vi "CRYReport Pic LIB.vi"(6 "sOption":string, 7 "sAction":string, 8 "nData":i32, 9 "sData":string, 10 "cView":T2, 11 "cFrame":T1) -> (0 "nData_Out":i32, 1 "sData_Out":string, 2 "cView_Out":T2, 3 "cFrame_Out":T1)   [LabVIEW 2013]
uses:
  CRYReport Global.vi
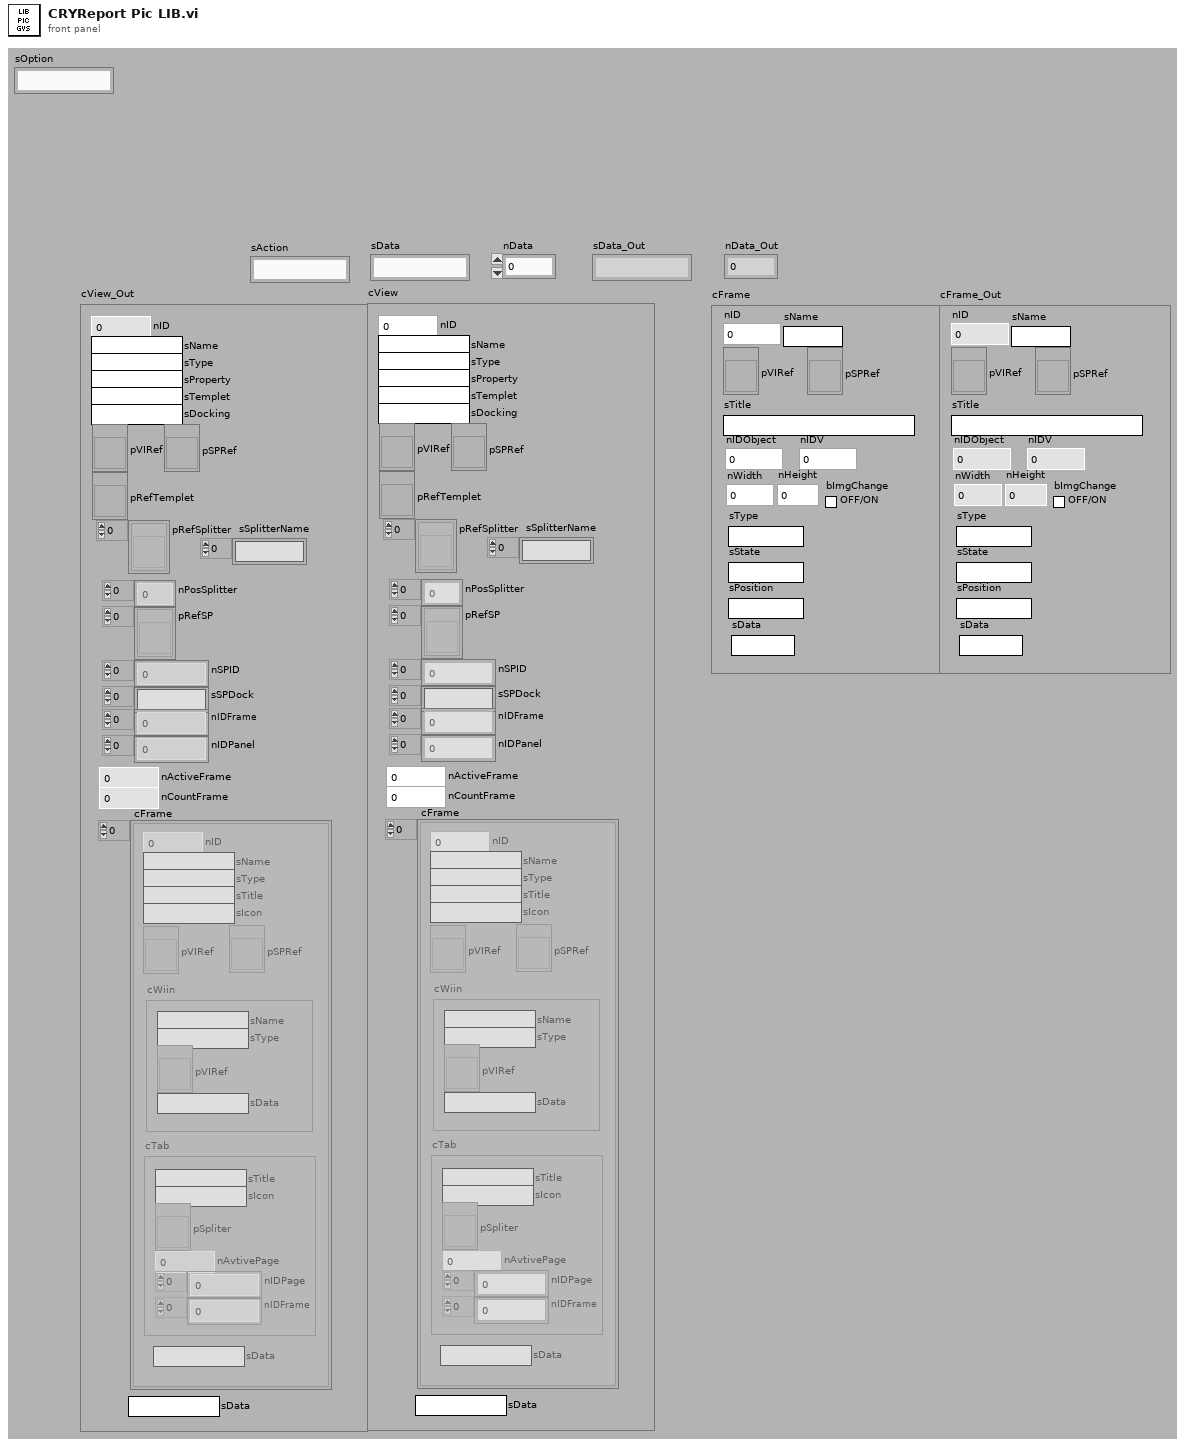
[diagram p1: front panel]
types:
  T1 = cluster{"nID":i16, "sName":string, "pVIRef":refnum<vi>, "pSPRef":refnum<vi>, "sTitle":string, "nIDObject":i16, "nIDV":i16, "nWidth":i16, "nHeight":i16, "bImgChange":bool, "sType":string, "sState":string, "sPosition":string, "sData":string}
  T2 = cluster{"nID":i32, "sName":string, "sType":string, "sProperty":string, "sTemplet":string, "sDocking":string, "pVIRef":refnum<vi>, "pSPRef":refnum<vi>, "pRefTemplet":refnum<vi>, "pRefSplitter":refnum<vi>[], "nPosSplitter":i32[], "pRefSP":refnum<vi>[], "nSPID":i32[], "sSPDock":string[], "nIDFrame":i32[], "nIDPanel":i32[], "nActiveFrame":i32, "nCountFrame":i32, "cFrame":cluster{"nID":i32, "sName":string, "sType":string, "sTitle":string, "sIcon":string, "pVIRef":refnum<vi>, "pSPRef":refnum<vi>, "cWiin":cluster{"sName":string, "sType":string, "pVIRef":refnum<vi>, "sData":string}, "cTab":cluster{"sTitle":string, "sIcon":string, "pSpliter":refnum<vi>, "nAvtivePage":i32, "nIDPage":i32[], "nIDFrame":i32[]}, "sData":string}[], "sData":string, "sSplitterName":string[]}
  T3 = enum16{"open", "replace", "create", "open or create", "replace or create", "replace or create with confirmation"}
  T4 = enum16{"big-endian, network order", "native, host order", "little-endian"}
  T5 = cluster{"nCount":i16, "cFrameList":cluster{"nID":i16, "sName":string, "pVIRef":refnum<vi>, "pSPRef":refnum<vi>, "sTitle":string, "nIDObject":i16, "nIDV":i16, "nWidth":i16, "nHeight":i16, "bImgChange":bool, "sType":string, "sState":string, "sPosition":string, "sData":string}[], "sData":string}
  T6 = typedef "LVRectTypeDef.ctl" = cluster{"Left":i16, "Top":i16, "Right":i16, "Bottom":i16}
  T7 = cluster{"nID":i16, "sName":string, "pVIRef":refnum<vi>, "pSPRef":refnum<vi>, "sTitle":string, "nIDObject":i16, "nIDV":i16, "nWidth":i16, "nHeight":i16, "bImgChange":bool, "sType":string, "sState":string, "sPosition":string, "sData":string}[]
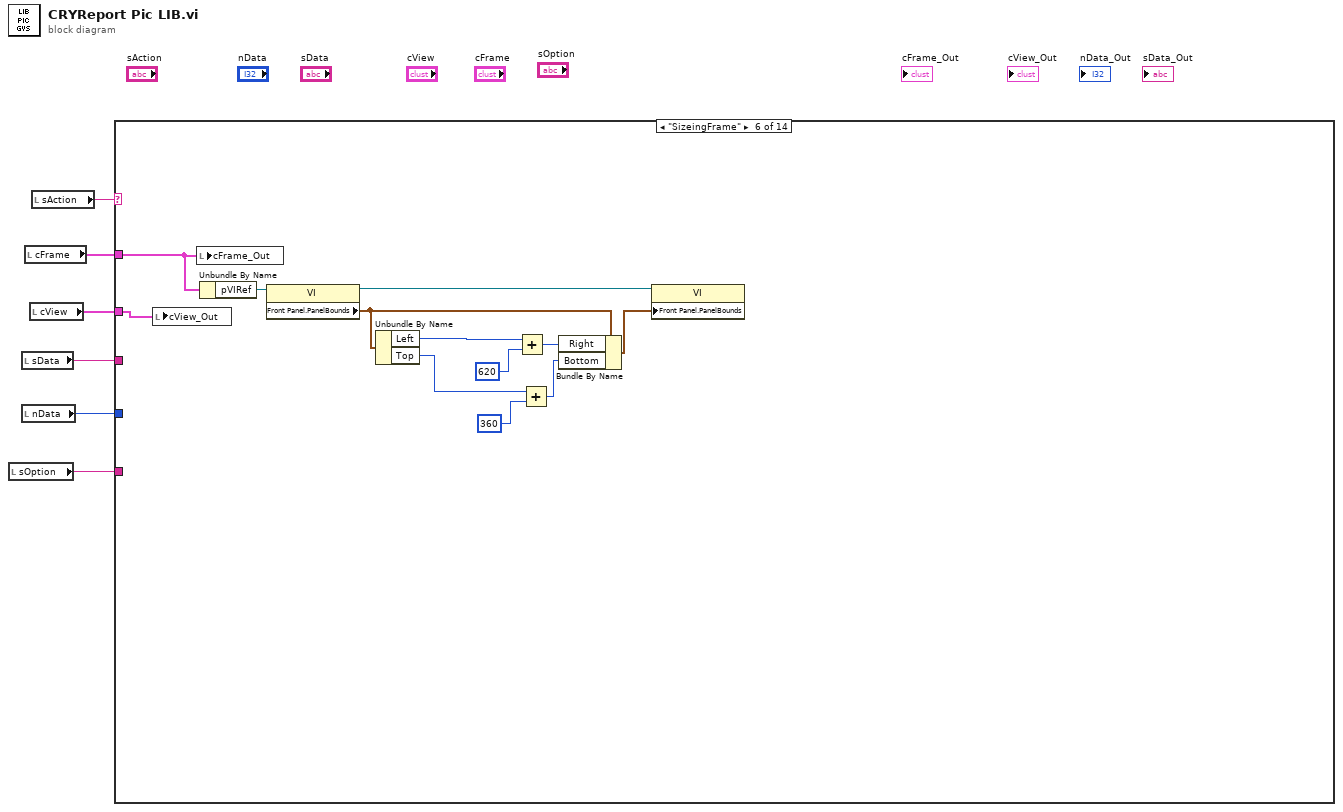
[diagram p0: block diagram]
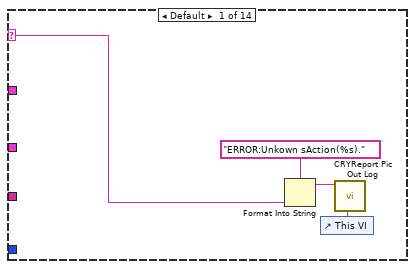
[diagram p2: hidden frame]
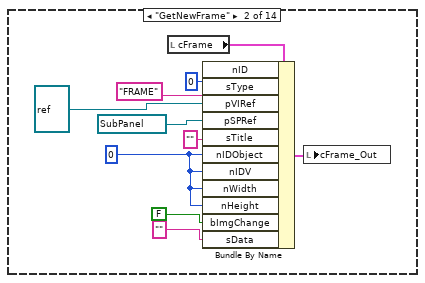
[diagram p3: hidden frame]
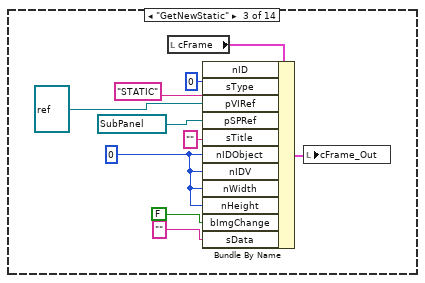
[diagram p4: hidden frame]
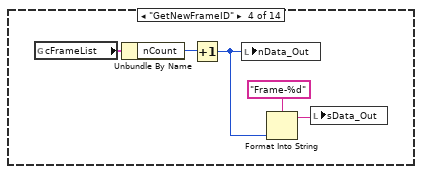
[diagram p5: hidden frame]
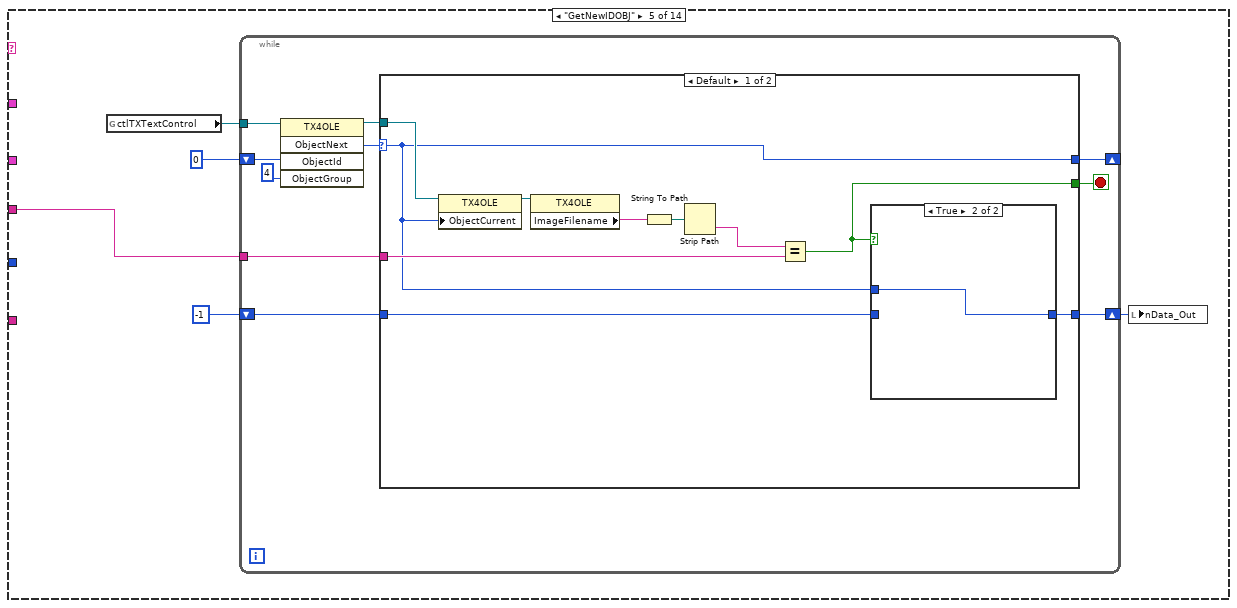
[diagram p6: hidden frame]
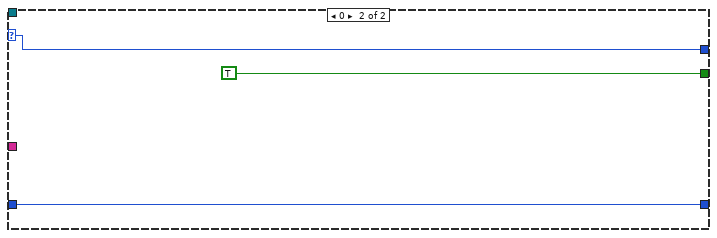
[diagram p8: hidden frame]
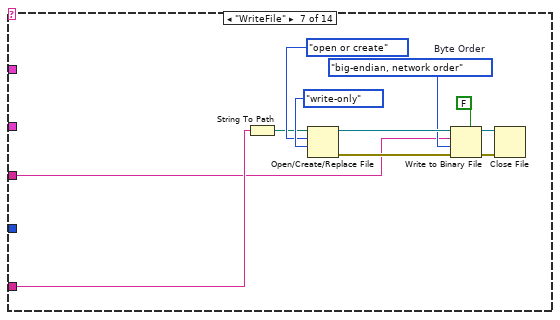
[diagram p9: hidden frame]
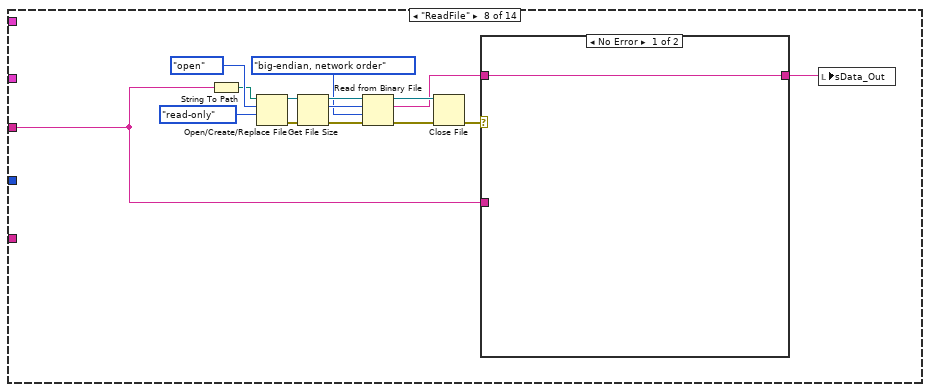
[diagram p10: hidden frame]
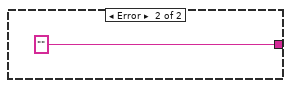
[diagram p11: hidden frame]
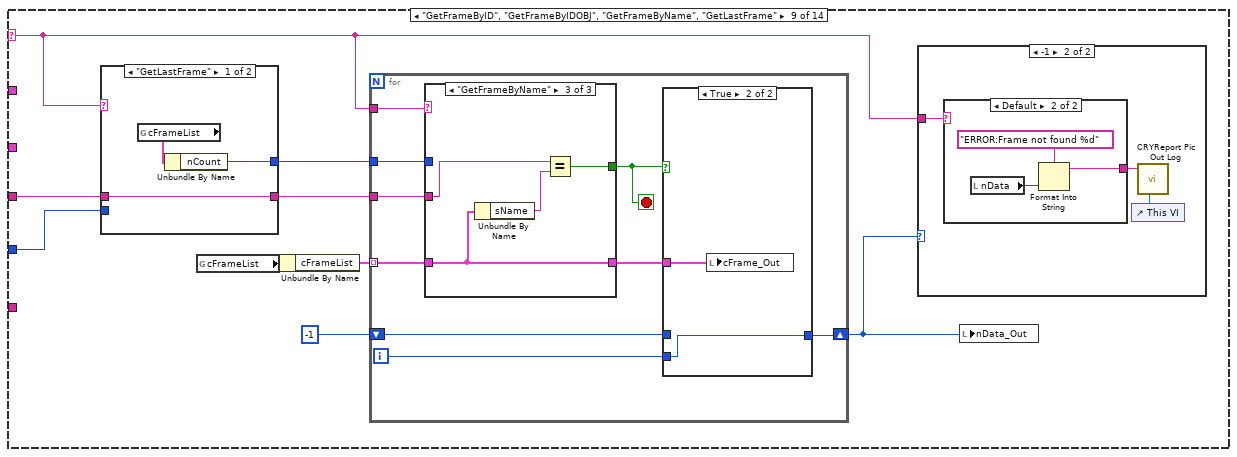
[diagram p12: hidden frame]
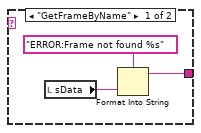
[diagram p14: hidden frame]
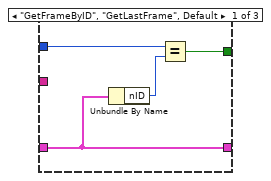
[diagram p17: hidden frame]
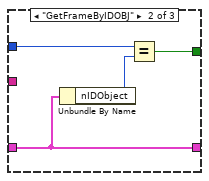
[diagram p18: hidden frame]
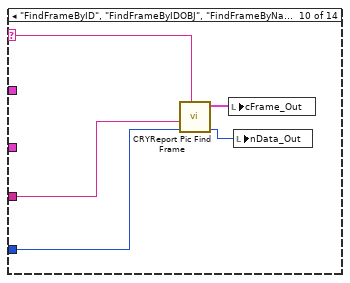
[diagram p19: hidden frame]
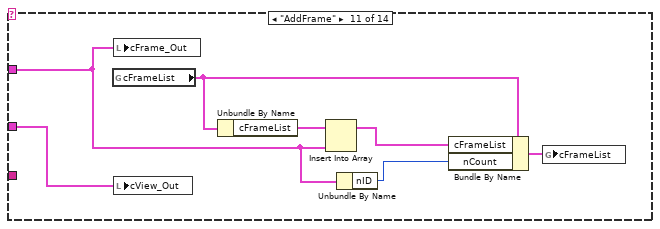
[diagram p20: hidden frame]
diagram:
  n1 = local read "sOption"() -> (w1:string)
  n2 = local read "sData"() -> (w5:string)
  n3 = local read "nData"() -> (w4:i32)
  n4 = local read "cFrame"() -> (w3:T1)
  n5 = local read "cView"() -> (w2:T2)
  n6 = local read "sAction"() -> (w6:string)
  n7 = case shown="\"SizeingFrame\"" w6 {
    selector: w6 -> [w8 _ _ _ _ _ _ _ w106 w157 _ _ _ _]
    tunnel: w5 -> [_ _ _ _ w38 _ w78 w89 w110 w156 _ _ _ _]
    tunnel: w4 -> [_ _ _ _ _ _ _ _ w113 w155 _ _ _ _]
    tunnel: w3 -> [_ _ _ _ _ w67 _ _ _ _ w159 w166 w183 _]
    tunnel: w2 -> [_ _ _ _ _ w66 _ _ _ _ w158 w169 w185 _]
    tunnel: w1 -> [_ _ _ _ _ _ w79 _ _ _ _ _ _ _]
    frame Default {
      n8 = Format Into String(format string="ERROR:Unkown sAction(%s).", w8) -> (resulting string=w7:string)  [unwired: 2 in, 1 out]
      n9 = control-ref of="This VI"() -> (w10:refnum<vi>)
      n10 = call "CRYReport Pic Out Log.vi"("vi reference"=w10, "sData"=w7) -> ()  [unwired: 10 in]
    }
    frame "GetNewFrame" {
      w17 = i16 0 ("nIDObject")
      n11 = local read "cFrame"() -> (w20:T1)
      n12 = Bundle By Name(cluster=w20, "nID"=i16 0, "sType"="FRAME", "pVIRef"=refnum<vi> refnum, "pSPRef"=refnum<vi> refnum, "sTitle"="", "nIDObject"=w17, "nIDV"=w17, "nWidth"=w17, "nHeight"=w17, "bImgChange"=FALSE, "sData"="") -> (w13:T1)
      n13 = local write "cFrame_Out"(w13) -> ()
    }
    frame "GetNewStatic" {
      w27 = i16 0 ("nIDObject")
      n14 = local read "cFrame"() -> (w30:T1)
      n15 = Bundle By Name(cluster=w30, "nID"=i16 0, "sType"="STATIC", "pVIRef"=refnum<vi> refnum, "pSPRef"=refnum<vi> refnum, "sTitle"="", "nIDObject"=w27, "nIDV"=w27, "nWidth"=w27, "nHeight"=w27, "bImgChange"=FALSE, "sData"="") -> (w23:T1)
      n16 = local write "cFrame_Out"(w23) -> ()
    }
    frame "GetNewFrameID" {
      n17 = global read "CRYReport Global.vi" "cFrameList"() -> (w34:T5)
      n18 = Unbundle By Name(w34) -> ("nCount"=w35:i16)
      n19 = Increment(x=w35) -> (x+1=w32:i16)
      n20 = local write "nData_Out"(w32) -> ()
      n21 = Format Into String(format string="Frame-%d", w32) -> (resulting string=w31:string)  [unwired: 2 in, 1 out]
      n22 = local write "sData_Out"(w31) -> ()
    }
    frame "GetNewIDOBJ" {
      n23 = global read "CRYReport Global.vi" "ctlTXTextControl"() -> (w40:refnum<k7>)
      n24 = while {
        tunnel: w40 -> [w50]
        shift-right: [w46] -> _
        shift-left: 0 -> [w49]
        tunnel: w38 -> [w43]
        shift-right: [w41] -> w36
        shift-left: -1 -> [w42]
        stop <- w45 stop-if-true
        n25 = invoke class="TX4OLE" method="ObjectNext"(reference=w50, "ObjectId"=w49, "ObjectGroup"=i16 4) -> (reference out=w44:refnum<k7>, "ObjectNext"=w47:i16)  [unwired: 2 in, 3 out]
        n26 = case shown="Default" w47 {
          selector: w47 -> [w54 w65]
          tunnel: [w54 w65] -> w46
          tunnel: [w57 TRUE] -> w45
          tunnel: w44 -> [w59 _]
          tunnel: w43 -> [w58 _]
          tunnel: w42 -> [w56 w63]
          tunnel: [w55 w63] -> w41
          frame Default {
            n27 = property class="TX4OLE"(reference=w59, "ObjectCurrent"=w54) -> (reference out=w60:refnum<k7>)  [unwired: 1 in, 1 out]
            n28 = property class="TX4OLE"(reference=w60) -> ("ImageFilename"=w51:string)  [unwired: 1 in, 2 out]
            n29 = String To Path(string=w51) -> (path=w52:path)
            n30 = Strip Path(path=w52) -> (name=w53:string)  [unwired: 1 out]
            n31 = Equal?(x=w53, y=w58) -> (x = y?=w57:bool)
            n32 = case shown="True" w57 {
              tunnel: [w61 w62] -> w55
              tunnel: w56 -> [w61 _]
              tunnel: w54 -> [_ w62]
              frame False {
              }
              frame True {
              }
            }
          }
          frame 0 {
          }
        }
      }
      n33 = local write "nData_Out"(w36) -> ()
    }
    frame "SizeingFrame" {
      n34 = local write "cView_Out"(w66) -> ()
      n35 = local write "cFrame_Out"(w67) -> ()
      n36 = Unbundle By Name(w67) -> ("pVIRef"=w77:refnum<vi>)
      n37 = property class="VI"(reference=w77) -> (reference out=w69:refnum<vi>, "Front Panel.PanelBounds"=w76:T6)  [unwired: 1 in, 1 out]
      n38 = Unbundle By Name(w76) -> ("Left"=w75:i16, "Top"=w70:i16)
      n39 = Add(x=w75, y=i16 620) -> (x+y=w72:i16)
      n40 = Add(x=w70, y=i16 360) -> (x+y=w71:i16)
      n41 = Bundle By Name(cluster=w76, "Right"=w72, "Bottom"=w71) -> (w68:T6)
      n42 = property class="VI"(reference=w69, "Front Panel.PanelBounds"=w68) -> ()  [unwired: 1 in, 2 out]
    }
    frame "WriteFile" {
      w85 = T4."big-endian, network order"  # Byte Order
      n43 = String To Path(string=w79) -> (path=w80:path)
      n44 = Open/Create/Replace File(file path (use dialog)=w80, operation (0:open)=T3."open or create", access (0:read/write)=enum16{"read/write", "read-only", "write-only"}."write-only") -> (refnum out=w88:refnum<file>, error out=w82:errorcluster)  [unwired: 1 in, 3 out]
      n45 = Write to Binary File(file (use dialog)=w88, data=w78, error in=w82, 5:FALSE ("prepend array or string size? (T)"), 9:w85) -> (refnum out=w83:refnum<file>, error out=w81:errorcluster)  [unwired: 2 out]
      n46 = Close File(refnum=w83, error in=w81) -> ()  [unwired: 2 out]
    }
    frame "ReadFile" {
      n47 = String To Path(string=w89) -> (path=w92:path)
      n48 = Open/Create/Replace File(file path (use dialog)=w92, operation (0:open)=T3."open", access (0:read/write)=enum16{"read/write", "read-only", "write-only"}."read-only") -> (refnum out=w99:refnum<file>, error out=w101:errorcluster)  [unwired: 1 in, 3 out]
      n49 = Get File Size(file=w99, error in=w101) -> (refnum out=w100:refnum<file>, size (in bytes)=w103:i64, 0:w102:errorcluster)
      n50 = Read from Binary File(8:w102, 9:T4."big-endian, network order" ("Byte Order"), 10:w103, 11:w100) -> (0:w98:errorcluster, 2:w91:string, 3:w97:refnum<file>)  [unwired: 3 out]
      n51 = Close File(refnum=w97, error in=w98) -> (error out=w93:errorcluster)  [unwired: 1 out]
      n52 = case shown="No Error" w93 {
        tunnel: w91 -> [w104 _]
        tunnel: [w104 ""] -> w90
        tunnel: w89 -> [_ _]
        frame No Error {
        }
        frame Error {
        }
      }
      n53 = local write "sData_Out"(w90) -> ()
    }
    frame "GetFrameByID", "GetFrameByIDOBJ", "GetFrameByName", "GetLastFrame" {
      n54 = case shown="\"GetLastFrame\"" w106 {
        tunnel: [w125 w128] -> w114
        tunnel: w113 -> [_ w128]
        tunnel: w110 -> [w124 w127]
        tunnel: [w124 w127] -> w109
        frame "GetLastFrame" {
          n55 = global read "CRYReport Global.vi" "cFrameList"() -> (w126:T5)
          n56 = Unbundle By Name(w126) -> ("nCount"=w125:i16)
        }
        frame "GetFrameByID", "GetFrameByIDOBJ", Default {
        }
      }
      n57 = global read "CRYReport Global.vi" "cFrameList"() -> (w112:T5)
      n58 = Unbundle By Name(w112) -> ("cFrameList"=w111:T7)
      n59 = for {
        tunnel: w114 -> [w136]
        tunnel: w111 -> [w135] mode=indexing
        tunnel: w106 -> [w137]
        tunnel: w109 -> [w132]
        shift-right: [w130] -> w107
        shift-left: -1 -> [w131]
        i -> [w129]
        stop <- w133 stop-if-true
        n60 = case shown="\"GetFrameByName\"" w137 {
          tunnel: w136 -> [w143 w147 _]
          tunnel: w135 -> [w141 w145 w150]
          tunnel: [w142 w146 w151] -> w133
          tunnel: [w141 w145 w150] -> w134
          tunnel: w132 -> [_ _ w149]
          frame "GetFrameByID", "GetLastFrame", Default {
            n61 = Unbundle By Name(w141) -> ("nID"=w144:i16)
            n62 = Equal?(x=w143, y=w144) -> (x = y?=w142:bool)
          }
          frame "GetFrameByIDOBJ" {
            n63 = Unbundle By Name(w145) -> ("nIDObject"=w148:i16)
            n64 = Equal?(x=w147, y=w148) -> (x = y?=w146:bool)
          }
          frame "GetFrameByName" {
            n65 = Unbundle By Name(w150) -> ("sName"=w152:string)
            n66 = Equal?(x=w149, y=w152) -> (x = y?=w151:bool)
          }
        }
        n67 = case shown="True" w133 {
          tunnel: w134 -> [_ w140]
          tunnel: w131 -> [w138 _]
          tunnel: [w138 w139] -> w130
          tunnel: w129 -> [_ w139]
          frame False {
          }
          frame True {
            n68 = local write "cFrame_Out"(w140) -> ()
          }
        }
      }
      n69 = case shown="-1" w107 {
        tunnel: w106 -> [_ w117]
        frame Default {
        }
        frame -1 {
          n70 = case shown="Default" w117 {
            tunnel: [w119 w121] -> w115
            frame "GetFrameByName" {
              n71 = local read "sData"() -> (w118:string)
              n72 = Format Into String(format string="ERROR:Frame not found %s", w118) -> (resulting string=w119:string)  [unwired: 2 in, 1 out]
            }
            frame Default {
              n73 = local read "nData"() -> (w122:i32)
              n74 = Format Into String(format string="ERROR:Frame not found %d", w122) -> (resulting string=w121:string)  [unwired: 2 in, 1 out]
            }
          }
          n75 = control-ref of="This VI"() -> (w116:refnum<vi>)
          n76 = call "CRYReport Pic Out Log.vi"("vi reference"=w116, "sData"=w115) -> ()  [unwired: 10 in]
        }
      }
      n77 = local write "nData_Out"(w107) -> ()
    }
    frame "FindFrameByID", "FindFrameByIDOBJ", "FindFrameByName" {
      n78 = call "CRYReport Pic Find Frame.vi"("sAction"=w157, "nData"=w155, "sData"=w156) -> ("nData_Out"=w153:i32, "cFrame_Out"=w154:T1)  [unwired: 7 in]
      n79 = local write "cFrame_Out"(w154) -> ()
      n80 = local write "nData_Out"(w153) -> ()
    }
    frame "AddFrame" {
      n81 = global read "CRYReport Global.vi" "cFrameList"() -> (w164:T5)
      n82 = local write "cFrame_Out"(w159) -> ()
      n83 = local write "cView_Out"(w158) -> ()
      n84 = Unbundle By Name(w164) -> ("cFrameList"=w163:T7)
      n85 = Insert Into Array(array=w163, new element=w159) -> (w162:T7)  [unwired: 1 in]
      n86 = Unbundle By Name(w159) -> ("nID"=w161:i16)
      n87 = Bundle By Name(cluster=w164, "cFrameList"=w162, "nCount"=w161) -> (w160:T5)
      n88 = global write "CRYReport Global.vi" "cFrameList"(w160) -> ()
    }
    frame "ReplaceFrame" {
      n89 = local write "cView_Out"(w169) -> ()
      n90 = local write "cFrame_Out"(w166) -> ()
      n91 = Unbundle By Name(w166) -> ("nID"=w167:i16)
      n92 = call "CRYReport Pic Find Frame.vi"("sAction"="FindFrameByID", "nData"=w167) -> ("nData_Out"=w165:i32)  [unwired: 8 in, 1 out]
      n93 = case shown="Default" w165 {
        tunnel: w165 -> [_ w176]
        tunnel: w166 -> [w171 w175]
        frame -1 {
          n94 = Unbundle By Name(w171) -> ("nID"=w170:i16)
          n95 = Format Into String(format string="ERROR:Frame not found %d", w170) -> (resulting string=w174:string)  [unwired: 2 in, 1 out]
          n96 = control-ref of="This VI"() -> (w173:refnum<vi>)
          n97 = call "CRYReport Pic Out Log.vi"("vi reference"=w173, "sData"=w174) -> ()  [unwired: 10 in]
        }
        frame Default {
          n98 = global read "CRYReport Global.vi" "cFrameList"() -> (w180:T5)
          n99 = Unbundle By Name(w180) -> ("cFrameList"=w179:T7)
          n100 = Replace Array Subset(array=w179, new element=w175, index=w176) -> (w178:T7)
          n101 = Bundle By Name(cluster=w180, "cFrameList"=w178) -> (w177:T5)
          n102 = global write "CRYReport Global.vi" "cFrameList"(w177) -> ()
        }
      }
    }
    frame "RemoveFrame" {
      n103 = local write "cView_Out"(w185) -> ()
      n104 = local write "cFrame_Out"(w183) -> ()
      n105 = Unbundle By Name(w183) -> ("nID"=w181:i16)
      n106 = call "CRYReport Pic Find Frame.vi"("sAction"="FindFrameByID", "nData"=w181) -> ("nData_Out"=w182:i32)  [unwired: 8 in, 1 out]
      n107 = case shown="Default" w182 {
        tunnel: w182 -> [_ w190]
        tunnel: w181 -> [w186 _]
        frame -1 {
          n108 = Format Into String(format string="ERROR:Frame not found %d", w186) -> (resulting string=w189:string)  [unwired: 2 in, 1 out]
          n109 = control-ref of="This VI"() -> (w188:refnum<vi>)
          n110 = call "CRYReport Pic Out Log.vi"("vi reference"=w188, "sData"=w189) -> ()  [unwired: 10 in]
        }
        frame Default {
          n111 = global read "CRYReport Global.vi" "cFrameList"() -> (w194:T5)
          n112 = Unbundle By Name(w194) -> ("cFrameList"=w193:T7)
          n113 = Delete From Array(array=w193, index=w190) -> (array with subset deleted=w192:T7)  [unwired: 1 in, 1 out]
          n114 = Bundle By Name(cluster=w194, "cFrameList"=w192) -> (w191:T5)
          n115 = global write "CRYReport Global.vi" "cFrameList"(w191) -> ()
        }
      }
    }
    frame "ClearTemp" {
      n116 = global read "CRYReport Global.vi" "pathTemp"() -> (w197:path)
      n117 = List Folder(path=w197) -> (path out=w195:path, filenames=w196:string[])  [unwired: 3 in, 2 out]
      n118 = for {
        tunnel: w196 -> [w200] mode=indexing
        tunnel: w195 -> [w201]
        n119 = Build Path(base path=w201, name or relative path=w200) -> (appended path=w199:path)
        n120 = Delete(path (use dialog)=w199) -> (error out=w198:errorcluster)  [unwired: 4 in, 2 out]
        n121 = case shown="No Error" w198 {
          frame No Error {
          }
          frame Error {
          }
        }
      }
    }
  }
